vi "Read Element of Guidance Array.vi"(8 "error in (no error)":errorcluster, 10 "index":i32, 11 "Vessel in":refnum<class "Vessel.lvclass">) -> (0 "error out":errorcluster, 2 "Guidance Library.lvlib:Guidance.lvclass":refnum<class "Guidance.lvclass">, 3 "Vessel out":refnum<class "Vessel.lvclass">)   [LabVIEW 2011, in "Vessel.lvclass"]
uses:
  Vessel.lvclass
  Guidance/Guidance.lvclass
  Vessel.lvclass/Vessel.ctl
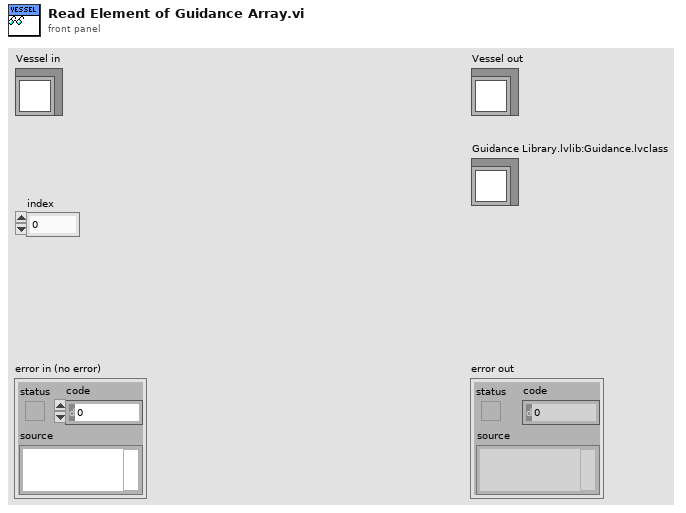
[diagram p1: front panel]
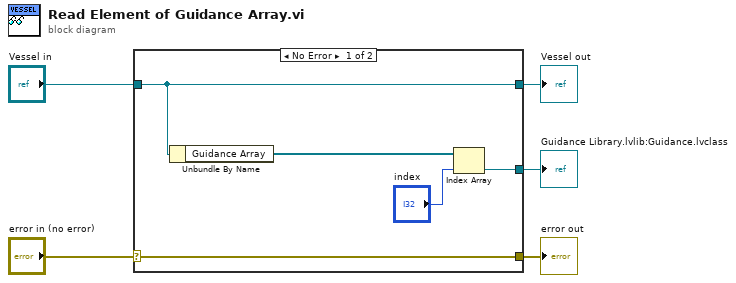
[diagram p0: block diagram]
diagram:
  n1 = case shown="No Error" "error in (no error)" {
    selector: "error in (no error)" -> [w10 w11]
    tunnel: [w10 w11] -> w4
    tunnel: [w9 w12] -> w2
    tunnel: "Vessel in" -> [w9 w12]
    tunnel: [w6 _] -> w1
    frame No Error {
      n2 = Unbundle By Name(w9) -> ("Guidance Array"=w8:refnum<class "Guidance.lvclass">[])
      n3 = Index Array(array=w8, index="index") -> (element=w6:refnum<class "Guidance.lvclass">)
    }
    frame Error {
    }
  }
  "error out" <- w4
  "Vessel out" <- w2
  "Guidance Library.lvlib:Guidance.lvclass" <- w1
